vi "Controller.vi"(8 "error in":errorcluster) -> ()   [LabVIEW 2014, in "Elevator System.lvlib"]
uses:
  Elevator System.lvlib
  Typedef/ControllerStates.ctl
  Typedef/Commands.ctl
  Typedef/MessageType.ctl
  Typedef/TeirNumber.ctl
  Typedef/ControllerStateData.ctl
  Typedef/StackCommandType.ctl
  Typedef/StackMessage.ctl
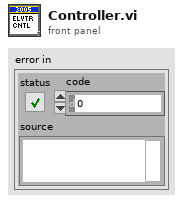
[diagram p1: front panel]
types:
  T1 = typedef "Elevator System.lvlib/ControllerStateData.ctl" = cluster{"State":T2, "Data":dbl}
  T2 = typedef "Elevator System.lvlib/ControllerStates.ctl" = enum16{"Init", "Set Elevator SP", "Set Gripper SP", "Wait For Elevator", "Wait For Gripper", ""}
  T3 = cluster{"Elevator":refnum<notifier>, "Gripper":refnum<notifier>}
  T4 = typedef "Elevator System.lvlib/MessageType.ctl" = cluster{"Name":T5, "Data":variant}
  T5 = typedef "Elevator System.lvlib/Commands.ctl" = enum16{"Home", "Stack", "Pickup", "Score", "Cycle", "Stop", "Manual Open", "Manual Close", "Manual Up", "Manual Down"}
  T6 = typedef "Elevator System.lvlib/StackMessage.ctl" = cluster{"Type":T7, "Teir":T8}
  T7 = typedef "Elevator System.lvlib/StackCommandType.ctl" = enum16{"Normal", "RC", "Step"}
  T8 = typedef "Elevator System.lvlib/TeirNumber.ctl" = enum16{"T1", "T2", "T3", "T4", "T5", "T6"}
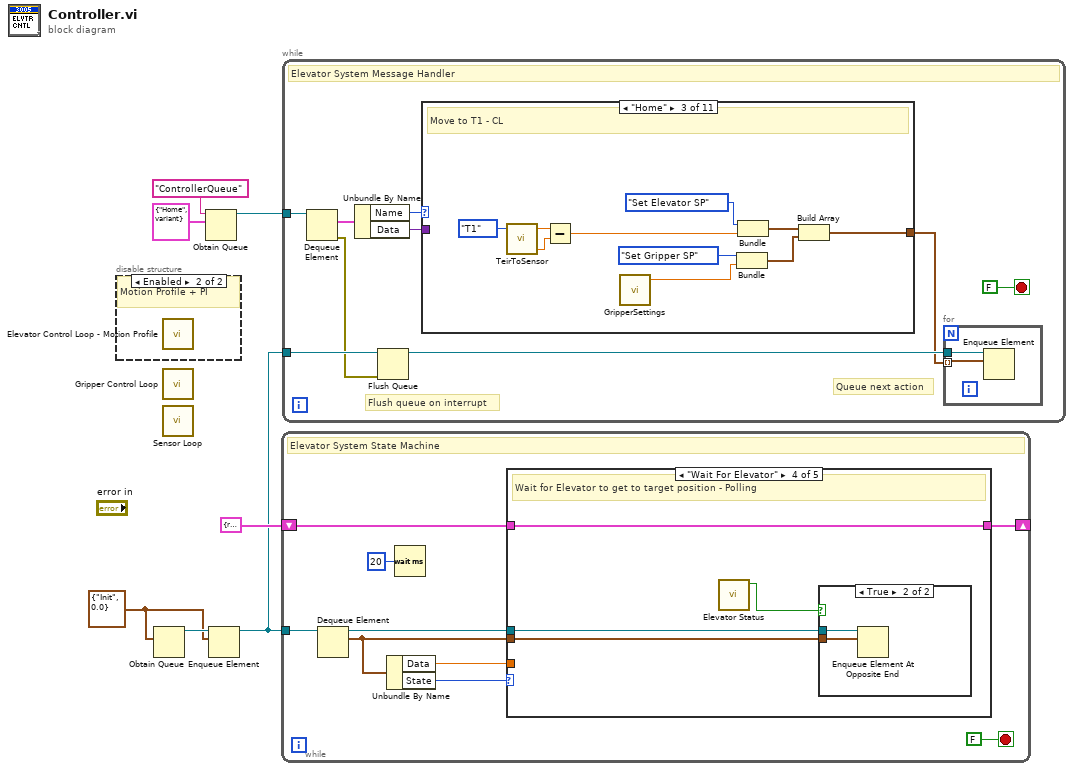
[diagram p0: block diagram]
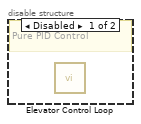
[diagram p2: hidden frame]
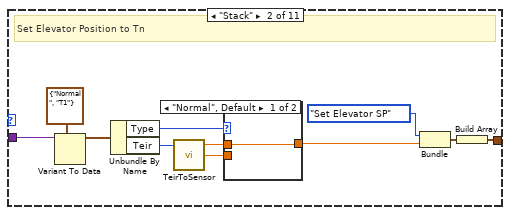
[diagram p4: hidden frame]
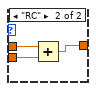
[diagram p5: hidden frame]
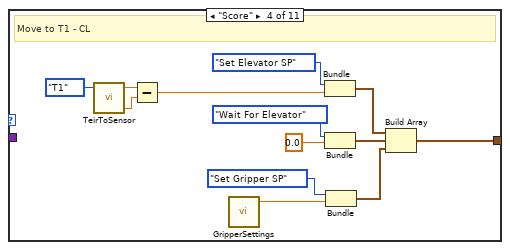
[diagram p6: hidden frame]
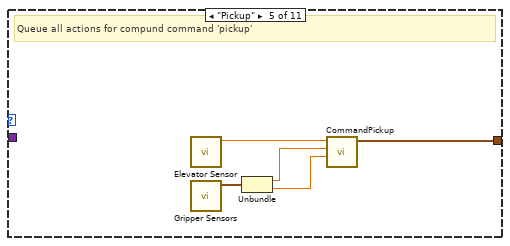
[diagram p7: hidden frame]
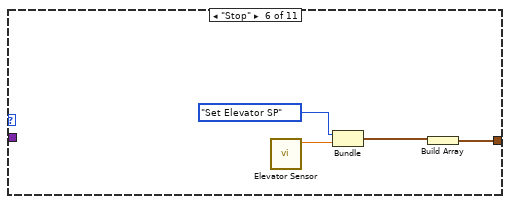
[diagram p8: hidden frame]
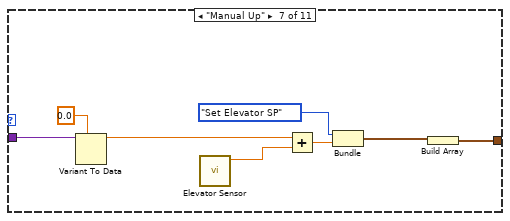
[diagram p9: hidden frame]
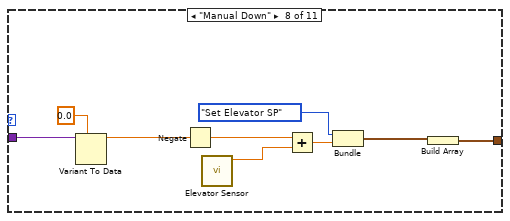
[diagram p10: hidden frame]
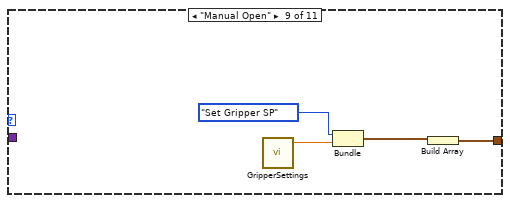
[diagram p11: hidden frame]
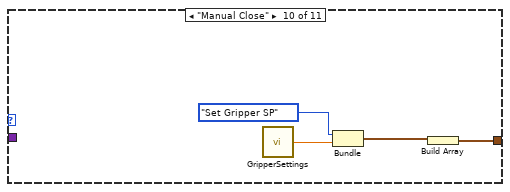
[diagram p12: hidden frame]
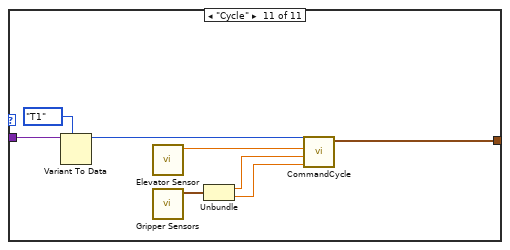
[diagram p13: hidden frame]
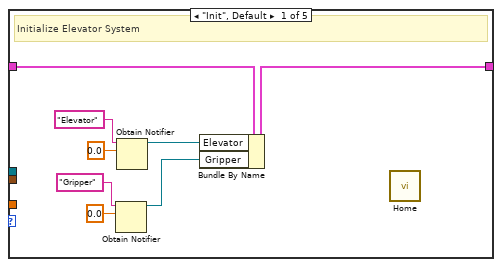
[diagram p14: hidden frame]
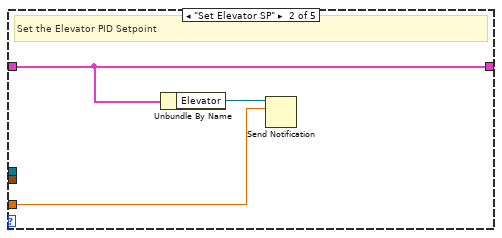
[diagram p15: hidden frame]
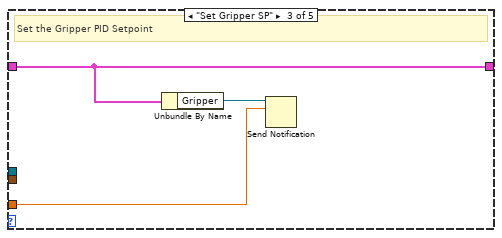
[diagram p16: hidden frame]
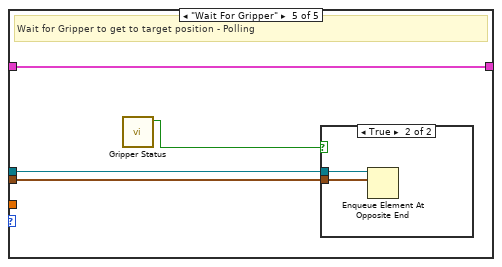
[diagram p18: hidden frame]
diagram:
  w1 = T1 {"State"=enum."Init", "Data"=0.0}
  n1 = disable-structure shown="Enabled" {
    frame Disabled {
      # "Pure PID Control"
      n2 = call "Elevator Control Loop.vi"() -> ()  [unwired: 12 in]
    }
    frame Enabled {
      # "Motion Profile + PI"
      n3 = call "Elevator Control Loop - Motion Profile.vi"() -> ()  [unwired: 12 in]
    }
  }
  n4 = Obtain Queue(element data type=w1) -> (queue out=w4:refnum<queue>)  [unwired: 4 in, 2 out]
  n5 = call "Gripper Control Loop.vi"() -> ()  [unwired: 12 in]
  n6 = call "Sensor Loop.vi"() -> ()  [unwired: 12 in]
  n7 = Obtain Queue(name (unnamed)="ControllerQueue", element data type=T4 {"Name"=enum."Home", "Data"=variant} ("Message")) -> (queue out=w5:refnum<queue>)  [unwired: 3 in, 2 out]
  n8 = Enqueue Element(queue=w4, element=w1) -> (queue out=w2:refnum<queue>)  [unwired: 2 in, 2 out]
  n9 = while {
    tunnel: w2 -> [w14]
    shift-right: [w9] -> _
    shift-left: T3 {"Elevator"=refnum, "Gripper"=refnum} -> [w10]
    stop <- FALSE stop-if-true
    # "Elevator System State Machine"
    n10 = Dequeue Element(queue=w14) -> (queue out=w13:refnum<queue>, element=w8:T1)  [unwired: 2 in, 2 out]
    n11 = Unbundle By Name(w8) -> ("Data"=w11:dbl, "State"=w12:T2)
    n12 = Wait (ms)(milliseconds to wait=u32 20) -> ()  [unwired: 1 out]
    n13 = case shown="\"Wait For Elevator\"" w12 {
      tunnel: w13 -> [_ _ _ w33 w38]
      tunnel: w11 -> [_ w25 w28 _ _]
      tunnel: w10 -> [w21 w27 w30 w34 w40]
      tunnel: [w20 w27 w30 w34 w40] -> w9
      tunnel: w8 -> [_ _ _ w32 w39]
      frame "Init", Default {
        # "Initialize Elevator System"
        n14 = Obtain Notifier(name (unnamed)="Gripper", notification data type=0.0 ("Setpoint")) -> (notifier out=w17:refnum<notifier>)  [unwired: 2 in, 2 out]
        n15 = Obtain Notifier(name (unnamed)="Elevator", notification data type=0.0 ("Setpoint")) -> (notifier out=w22:refnum<notifier>)  [unwired: 2 in, 2 out]
        n16 = Bundle By Name(cluster=w21, "Elevator"=w22, "Gripper"=w17) -> (w20:T3)
        n17 = call "Home.vi"() -> ()  [unwired: 12 in]
      }
      frame "Set Elevator SP" {
        # "Set the Elevator PID Setpoint"
        n18 = Unbundle By Name(w27) -> ("Elevator"=w26:refnum<notifier>)
        n19 = Send Notification(notification=w25, notifier=w26) -> ()  [unwired: 1 in, 2 out]
      }
      frame "Set Gripper SP" {
        # "Set the Gripper PID Setpoint"
        n20 = Unbundle By Name(w30) -> ("Gripper"=w29:refnum<notifier>)
        n21 = Send Notification(notification=w28, notifier=w29) -> ()  [unwired: 1 in, 2 out]
      }
      frame "Wait For Elevator" {
        # "Wait for Elevator to get to target position - Polling"
        n22 = call "Elevator Status.vi"() -> ("Moving?"=w31:bool)  [unwired: 9 in, 2 out]
        n23 = case shown="True" w31 {
          tunnel: w33 -> [_ w36]
          tunnel: w32 -> [_ w35]
          frame False {
          }
          frame True {
            n24 = Enqueue Element At Opposite End(queue=w36, element=w35) -> ()  [unwired: 2 in, 3 out]
          }
        }
      }
      frame "Wait For Gripper" {
        # "Wait for Gripper to get to target position - Polling"
        n25 = call "Gripper Status.vi"() -> ("Moving?"=w37:bool)  [unwired: 9 in, 2 out]
        n26 = case shown="True" w37 {
          tunnel: w38 -> [_ w42]
          tunnel: w39 -> [_ w41]
          frame False {
          }
          frame True {
            n27 = Enqueue Element At Opposite End(queue=w42, element=w41) -> ()  [unwired: 2 in, 3 out]
          }
        }
      }
    }
  }
  n28 = while {
    tunnel: w5 -> [w47]
    tunnel: w2 -> [w48]
    stop <- FALSE stop-if-true
    # "Queue next action"
    # "Flush queue on interrupt"
    # "Elevator System Message Handler"
    n29 = Dequeue Element(queue=w47) -> (element=w46:T4, error out=w43:errorcluster)  [unwired: 2 in, 2 out]
    n30 = Unbundle By Name(w46) -> ("Name"=w50:T5, "Data"=w49:variant)
    n31 = Flush Queue(queue=w48, error in (no error)=w43) -> (queue out=w51:refnum<queue>)  [unwired: 2 out]
    n32 = case shown="\"Home\"" w50 {
      tunnel: w49 -> [_ w62 _ _ _ _ w102 w111 _ _ w130]
      tunnel: [_ w59 w74 w87 w94 w96 w104 w113 w116 w121 w131] -> w45
      frame Default {
      }
      frame "Stack" {
        # "Set Elevator Position to Tn"
        n33 = Variant To Data(type=T6 {"Type"=enum."Normal", "Teir"=enum."T1"}, Variant=w62) -> (data=w57:T6)  [unwired: 1 in, 1 out]
        n34 = Unbundle By Name(w57) -> ("Type"=w52:T7, "Teir"=w56:T8)
        n35 = call "TeirToSensor.vi"("Teir"=w56) -> ("CR"=w54:dbl, "Teir Height"=w55:dbl)  [unwired: 2 in, 1 out]
        n36 = case shown="\"Normal\", Default" w52 {
          tunnel: w55 -> [w63 w66]
          tunnel: w54 -> [_ w65]
          tunnel: [w63 w64] -> w53
          frame "Normal", Default {
          }
          frame "RC" {
            n37 = Add(x=w66, y=w65) -> (x+y=w64:dbl)
          }
        }
        n38 = Bundle("States"=ControllerStates."Set Elevator SP", "Teir Height"=w53) -> (w60:cluster{"States":T2, "Teir Height":dbl})  [unwired: 1 in]
        n39 = Build Array(w60) -> (w59:cluster{"States":T2, "Teir Height":dbl}[])
      }
      frame "Home" {
        # "Move to T1 - CL"
        n40 = call "TeirToSensor.vi"("Teir"=TeirNumber."T1" ("Enum")) -> ("CL"=w71:dbl, "Teir Height"=w72:dbl)  [unwired: 2 in, 1 out]
        n41 = Subtract(x=w72, y=w71) -> (x-y=w68:dbl)
        n42 = call "GripperSettings.vi"() -> ("Open"=w67:dbl)  [unwired: 2 in, 2 out]
        n43 = Bundle("States"=ControllerStates."Set Gripper SP", "Open"=w67) -> (w69:cluster{"States":T2, "Open":dbl})  [unwired: 1 in]
        n44 = Bundle("States"=ControllerStates."Set Elevator SP", w68) -> (w75:cluster{"States":T2, dbl})  [unwired: 1 in]
        n45 = Build Array(w75, w69) -> (w74:cluster{"States":T2, "Open":dbl}[])
      }
      frame "Score" {
        # "Move to T1 - CL"
        n46 = call "TeirToSensor.vi"("Teir"=TeirNumber."T1" ("Enum")) -> ("CL"=w84:dbl, "Teir Height"=w85:dbl)  [unwired: 2 in, 1 out]
        n47 = Subtract(x=w85, y=w84) -> (x-y=w81:dbl)
        n48 = call "GripperSettings.vi"() -> ("Open"=w80:dbl)  [unwired: 2 in, 2 out]
        n49 = Bundle("States"=ControllerStates."Set Elevator SP", w81) -> (w88:cluster{"States":T2, dbl})  [unwired: 1 in]
        n50 = Bundle("States"=ControllerStates."Wait For Elevator", 0.0) -> (w78:cluster{"States":T2, dbl})  [unwired: 1 in]
        n51 = Bundle("States"=ControllerStates."Set Gripper SP", "Open"=w80) -> (w82:cluster{"States":T2, "Open":dbl})  [unwired: 1 in]
        n52 = Build Array(w88, w78, w82) -> (w87:cluster{"States":T2, "Open":dbl}[])
      }
      frame "Pickup" {
        # "Queue all actions for compund command 'pickup'"
        n53 = call "Elevator Sensor.vi"() -> ("Value"=w92:dbl)  [unwired: 10 in, 1 out]
        n54 = call "Gripper Sensors.vi"() -> ("Gripper Values"=w93:cluster{"Left":dbl, "Right":dbl})  [unwired: 10 in, 1 out]
        n55 = Unbundle(w93) -> ("Left"=w90:dbl, "Right"=w91:dbl)
        n56 = call "CommandPickup.vi"("Gripper Value R"=w91, "Gripper Value L"=w90, "Elevator Value"=w92) -> ("appended array"=w94:cluster{"States":T2, "Numeric":dbl}[])  [unwired: 8 in]
      }
      frame "Stop" {
        n57 = call "Elevator Sensor.vi"() -> ("Value"=w95:dbl)  [unwired: 10 in, 1 out]
        n58 = Bundle("States"=ControllerStates."Set Elevator SP", "Value"=w95) -> (w97:cluster{"States":T2, "Value":dbl})  [unwired: 1 in]
        n59 = Build Array(w97) -> (w96:cluster{"States":T2, "Value":dbl}[])
      }
      frame "Manual Up" {
        n60 = Variant To Data(type=0.0, Variant=w102) -> (data=w100:dbl)  [unwired: 1 in, 1 out]
        n61 = call "Elevator Sensor.vi"() -> ("Value"=w99:dbl)  [unwired: 10 in, 1 out]
        n62 = Add(x=w100, y=w99) -> (x+y=w103:dbl)
        n63 = Bundle("States"=ControllerStates."Set Elevator SP", w103) -> (w105:cluster{"States":T2, dbl})  [unwired: 1 in]
        n64 = Build Array(w105) -> (w104:cluster{"States":T2, dbl}[])
      }
      frame "Manual Down" {
        n65 = Variant To Data(type=0.0, Variant=w111) -> (data=w109:dbl)  [unwired: 1 in, 1 out]
        n66 = Negate(x=w109) -> (-x=w108:dbl)
        n67 = call "Elevator Sensor.vi"() -> ("Value"=w107:dbl)  [unwired: 10 in, 1 out]
        n68 = Add(x=w108, y=w107) -> (x+y=w112:dbl)
        n69 = Bundle("States"=ControllerStates."Set Elevator SP", w112) -> (w114:cluster{"States":T2, dbl})  [unwired: 1 in]
        n70 = Build Array(w114) -> (w113:cluster{"States":T2, dbl}[])
      }
      frame "Manual Open" {
        n71 = call "GripperSettings.vi"() -> ("Open"=w117:dbl)  [unwired: 2 in, 2 out]
        n72 = Bundle("States"=ControllerStates."Set Gripper SP", "Open"=w117) -> (w118:cluster{"States":T2, "Open":dbl})  [unwired: 1 in]
        n73 = Build Array(w118) -> (w116:cluster{"States":T2, "Open":dbl}[])
      }
      frame "Manual Close" {
        n74 = call "GripperSettings.vi"() -> ("Close"=w120:dbl)  [unwired: 2 in, 2 out]
        n75 = Bundle("States"=ControllerStates."Set Gripper SP", "Close"=w120) -> (w122:cluster{"States":T2, "Close":dbl})  [unwired: 1 in]
        n76 = Build Array(w122) -> (w121:cluster{"States":T2, "Close":dbl}[])
      }
      frame "Cycle" {
        n77 = Variant To Data(type=TeirNumber."T1" ("data"), Variant=w130) -> (data=w128:T8)  [unwired: 1 in, 1 out]
        n78 = call "Elevator Sensor.vi"() -> ("Value"=w126:dbl)  [unwired: 10 in, 1 out]
        n79 = call "Gripper Sensors.vi"() -> ("Gripper Values"=w127:cluster{"Left":dbl, "Right":dbl})  [unwired: 10 in, 1 out]
        n80 = Unbundle(w127) -> ("Left"=w125:dbl, "Right"=w124:dbl)
        n81 = call "CommandCycle.vi"("Gripper Value R"=w124, "Gripper Value L"=w125, "Elevator Value"=w126, "Teir Selection"=w128) -> ("appended array"=w131:cluster{"States":T2, "Numeric":dbl}[])  [unwired: 7 in]
      }
    }
    n82 = for {
      tunnel: w51 -> [w133]
      tunnel: w45 -> [w132] mode=indexing
      n83 = Enqueue Element(queue=w133, element=w132) -> ()  [unwired: 2 in, 3 out]
    }
  }
